vi "SENS_CORR_EXT_AUTO_STAR.vi"(0 "VISA IN":refnum<visa-resource-name>, 1 "Start Frq.":i32, 5 "error in":errorcluster, 7 "Channel":i32) -> (14 "VISA Out":refnum<visa-resource-name>, 19 "error out":errorcluster)   [LabVIEW 2018, in "PNA-X.lvlib"]
doc: "SENSe<cnum>:CORRection:EXTension:AUTO:STARt <value> \n(Read-Write) Set the start frequency for custom user span. Learn more about User Span. \nParameters \n<cnum> Any existing channel number. If unspecified, value is set to 1 \n<value> User span start value. Must be within the frequency range of the active channel \nand less than the value set by SENS:CORR:EXT:AUTO:STOP. \nExamples SENS:CORR:EXT:AUTO:STAR 1E9 \nsense2:correction:extension:auto:start 200e6 \nQuery Syntax SENSe<cnum>:CORRection:EXTension:AUTO:STARt <value>? \nReturn Type Numeric \nDefault Start frequency of the current active channel."
uses:
  PNA-X.lvlib
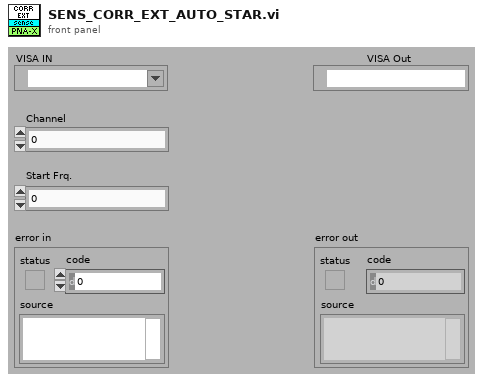
[diagram p1: front panel]
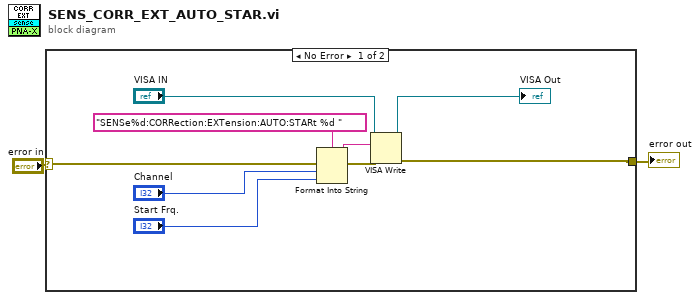
[diagram p0: block diagram]
diagram:
  n1 = case shown="No Error" "error in" {
    selector: "error in" -> [w11 w12]
    tunnel: [w6 w12] -> w1
    frame No Error {
      n2 = Format Into String(format string="SENSe%d:CORRection:EXTension:AUTO:STARt %d " ("Cmdline"), error in=w11, "Channel", "Start Frq.") -> (resulting string=w9:string, error out=w10:errorcluster)  [unwired: 1 in]
      n3 = VISA Write(VISA resource name="VISA IN", write buffer=w9, error in (no error)=w10) -> (VISA resource name out=→"VISA Out":refnum<visa-resource-name>, error out=w6:errorcluster)  [unwired: 1 out]
    }
    frame Error {
    }
  }
  "error out" <- w1
